vi "USB3 Requeue Buffer.vi"(8 "error in (no error)":errorcluster, 10 "hBuffer":u64, 11 "hCamera":u64) -> (0 "error out":errorcluster, 1 "function return":i32, 2 "hBuffer out":u64, 3 "hCamera out":u64)   [LabVIEW 2013, in "Octoplus_LIDAR.lvlib"]
doc: "CAMCMOSOCTUSB3_API int __cdecl USB3_RequeueBuffer(CAM_HANDLE hCamera, BUFF_HANDLE hBuffer);"
uses:
  <userlib>/Octoplus_LIDAR/Octoplus_LIDAR.lvlib
  <userlib>/Octoplus_LIDAR/CamCmosOctUsb3.dll
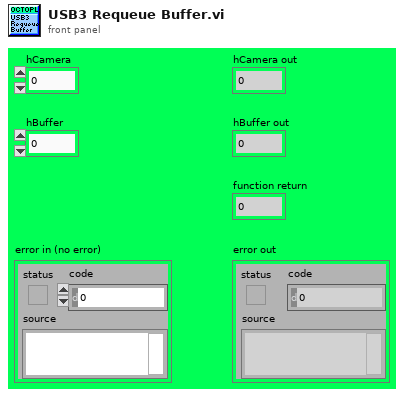
[diagram p1: front panel]
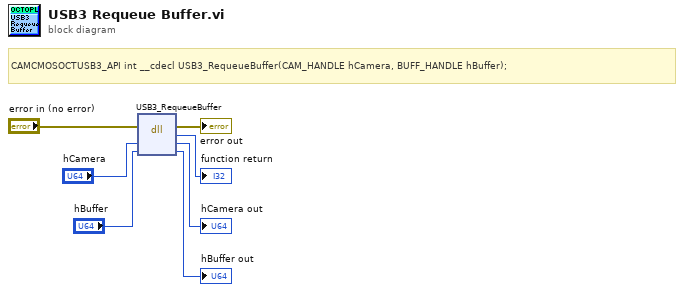
[diagram p0: block diagram]
diagram:
  # "CAMCMOSOCTUSB3_API int __cdecl USB3_RequeueBuffer(CAM_HANDLE hCamera, BUFF_HANDLE hBuffer);"
  n1 = dll-call lib="C:/Program Files/National Instruments/LabVIEW 2013/user.lib/Octoplus_LIDAR/CamCmosOctUsb3.*" fn="USB3_RequeueBuffer"(error in="error in (no error)", "hCamera"="hCamera", "hBuffer"="hBuffer") -> (error out=→"error out":errorcluster, "return type"=→"function return":i32, "hCamera"=→"hCamera out":u64, "hBuffer"=→"hBuffer out":u64)  [unwired: 2 in, 1 out]
